vi "Load XCL template.vi"(10 "Measurement template file":path, 11 "Measurement properties":T1={"Measurement frequencies (Hz)"=[1000.0, 10000.0, 1000.0], "Sampling frequency (Hz)"=500000.0, "Signal amplitude (V)"=4.5, "AC-DC settle time (s)"=20.0, "Record length (multiples of period)"=[1000.0, 10000.0, 1000.0], "Measurement template file"=path "", "Row of START keyword"=0, "Row of STOP keyword"=0, "Calculate RMS from samples"=FALSE, "AC-DC warm up time (s)"=300.0} {"Record length (multiples of period)" format="%#_3p"; "Sampling frequency (Hz)" format="%#_3p"; "Measurement frequencies (Hz)" format="%#_3p"}) -> (3 "Measurement properties out":T1={"Measurement frequencies (Hz)"=[1000.0, 10000.0, 1000.0], "Sampling frequency (Hz)"=500000.0, "Signal amplitude (V)"=4.5, "AC-DC settle time (s)"=20.0, "Record length (multiples of period)"=[1000.0, 10000.0, 1000.0], "Measurement template file"=path "", "Row of START keyword"=0, "Row of STOP keyword"=0, "Calculate RMS from samples"=FALSE, "AC-DC warm up time (s)"=300.0} {"Record length (multiples of period)" format="%#_3p"; "Sampling frequency (Hz)" format="%#_3p"; "Measurement frequencies (Hz)" format="%#_3p"})   [LabVIEW 2020]
doc: "Reads values from measurement template in excell spreadsheet."
uses:
  Measurement/Type definitions/Measuement properties.ctl
  <vilib>/Utility/NIReport.llb/Report Type.ctl
  <vilib>/Utility/error.llb/DialogType.ctl
  <vilib>/addons/_office/excel.llb/Excel Get Data ([str]).vi
  <vilib>/Utility/NIReport.llb/NI_report.lvclass
  <vilib>/addons/_office/NI_ReportGenerationToolkit.lvlib
  <vilib>/Utility/NIReport.llb/NI_ReportGenerationCore.lvlib
  <vilib>/Utility/NIReport.llb/Excel/NI_Excel.lvclass
panel:
  out "Stop row":i32
  out "Start row":i32
  out "excell template content":string[][](array[string])
  out "error out":errorcluster
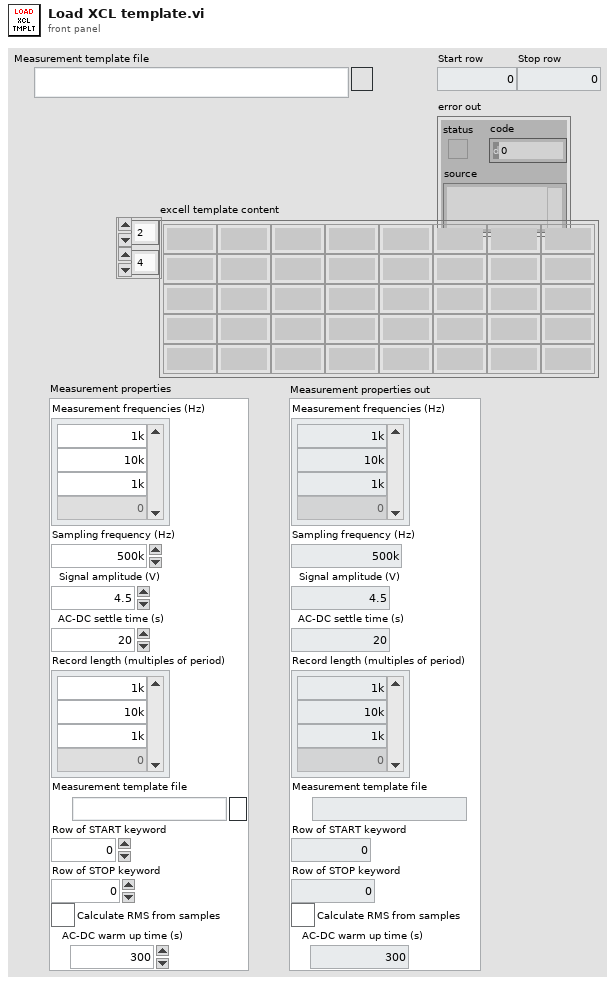
[diagram p1: front panel]
types:
  T1 = typedef "Measuement properties.ctl" = cluster{"Measurement frequencies (Hz)":dbl[], "Sampling frequency (Hz)":dbl, "Signal amplitude (V)":dbl, "AC-DC settle time (s)":dbl, "Record length (multiples of period)":dbl[], "Measurement template file":path, "Row of START keyword":i32, "Row of STOP keyword":i32, "Calculate RMS from samples":bool, "AC-DC warm up time (s)":dbl}
  T2 = enum16{"maximized", "minimized", "normal", "no change"}
  T3 = typedef "NI_ReportGenerationCore.lvlib/Report Type.ctl" = enum16{"HTML", "Word", "Excel"}
  T4 = typedef "DialogType.ctl" = u16
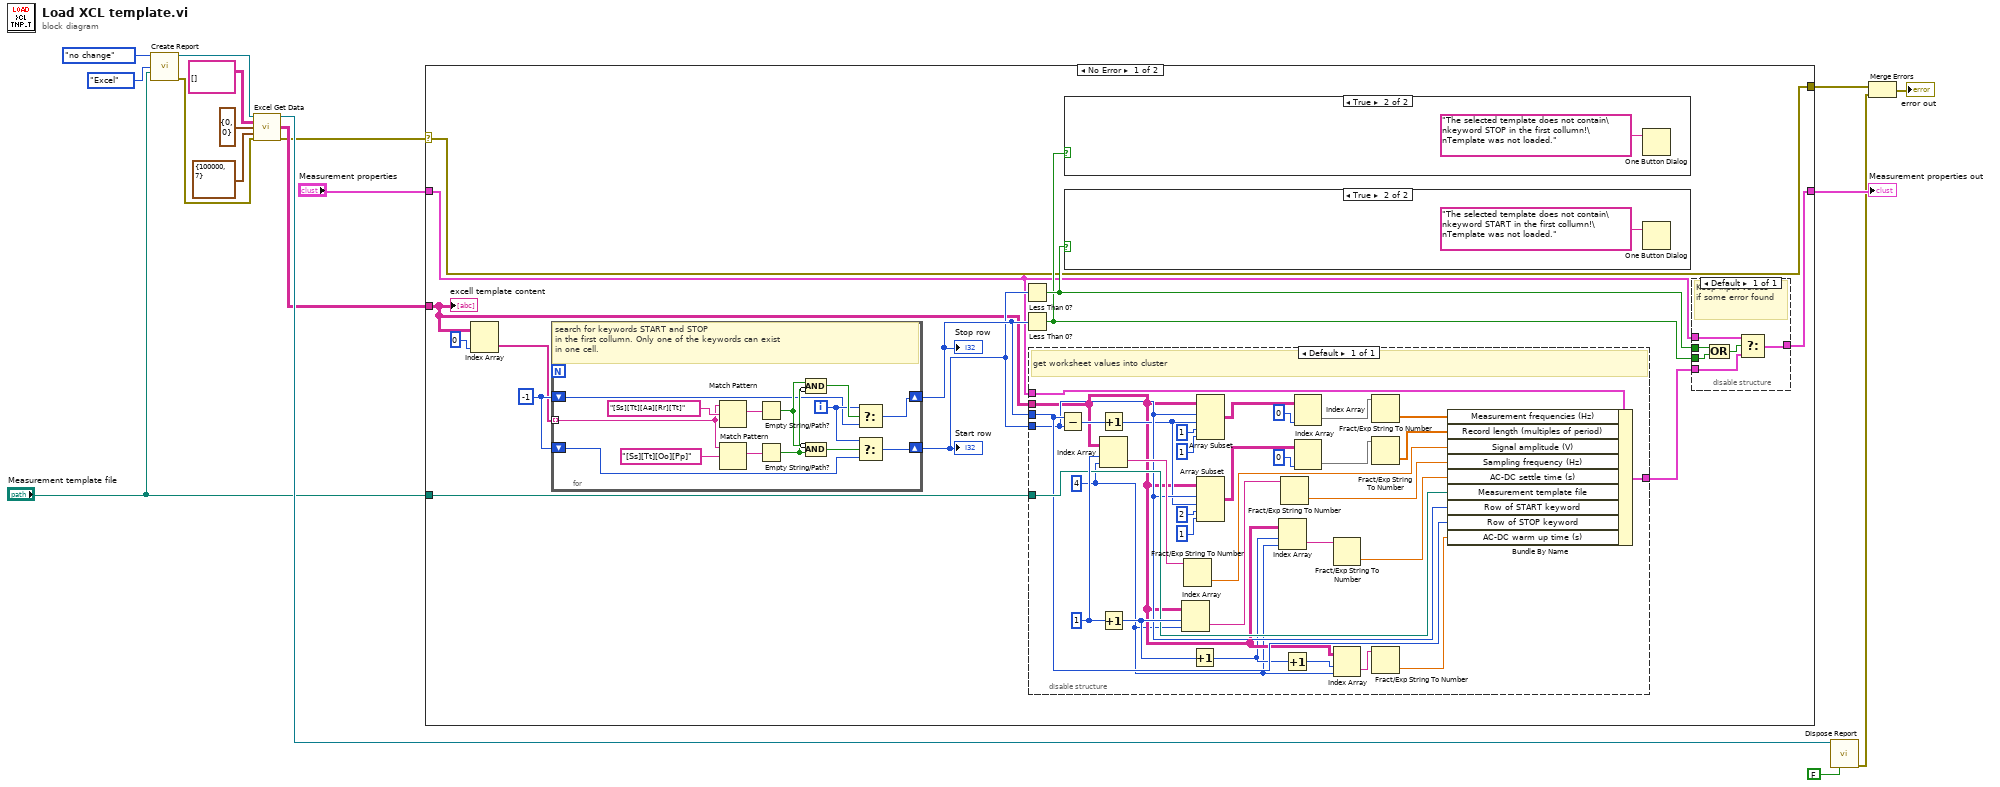
[diagram p0: block diagram]
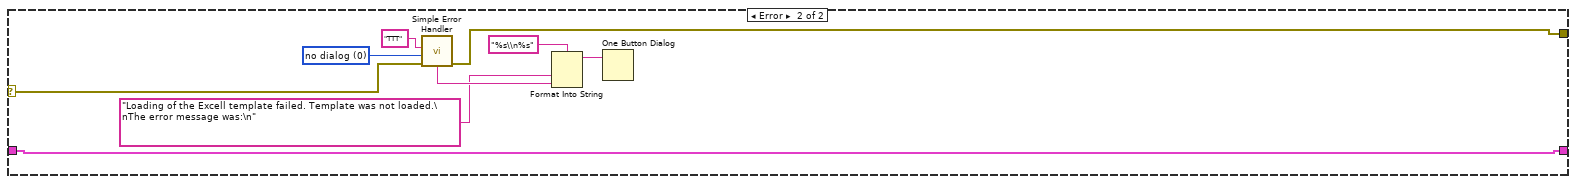
[diagram p4: hidden frame]
diagram:
  n1 = call <vilib>:"Create Report.vi"("window state (normal)"=T2."no change", "report type"=Report_Type."Excel", "template (empty)"="Measurement template file") -> ("report out"=w17:refnum<class "NI_report.lvclass">, "error out"=w16:errorcluster)  [unwired: 11 in]
  n2 = call-poly <vilib>:"Excel Get Data.vi"("report in"=w17, "data type"=string[][] [], "start (-1, -1)"=cluster{"row":i32, "column":i32} {"row"=0, "column"=0}, "end (-1, -1)"=cluster{"row":i32, "column":i32} {"row"=100000, "column"=7}, "error in (no error)"=w16) -> ("report out"=w15:refnum<class "NI_report.lvclass">, "data"=w11:string[][], "error out"=w4:errorcluster)  [unwired: 8 in]
  n3 = case shown="No Error" w4 {
    selector: w4 -> [w18 w93]
    tunnel: w11 -> [w25 _]
    tunnel: [w21 w94] -> w10
    tunnel: "Measurement properties" -> [w20 w94]
    tunnel: "Measurement template file" -> [w19 _]
    tunnel: [w18 w90] -> w3
    frame No Error {
      w29 = -1
      n4 = Index Array(array=w25, index (col)=0 ("disabled index (col)")) -> (element=w28:string[])  [unwired: 1 in]
      n5 = for {
        tunnel: w28 -> [w84] mode=indexing
        shift-right: [w79] -> w26
        shift-left: w29 -> [w72]
        shift-right: [w74] -> w27
        shift-left: w29 -> [w73]
        i -> [w75]
        # "search for keywords START and STOP\nin the first collumn. Only one of the keywords can exist\nin one cell."
        n6 = Match Pattern(string=w84, regular expression="[Ss][Tt][Aa][Rr][Tt]") -> (match substring=w82:string)  [unwired: 1 in, 3 out]
        n7 = Match Pattern(string=w84, regular expression="[Ss][Tt][Oo][Pp]") -> (match substring=w81:string)  [unwired: 1 in, 3 out]
        n8 = Empty String/Path?(string/path=w82) -> (empty?=w78:bool)
        n9 = Empty String/Path?(string/path=w81) -> (empty?=w77:bool)
        n10 = Compound Arithmetic op=AND(w78, invert w77) -> (w76:bool)
        n11 = Compound Arithmetic op=AND(invert w78, w77) -> (w80:bool)
        n12 = Select(t=w75, s=w76, f=w73) -> (s? t:f=w74:i32)
        n13 = Select(t=w75, s=w80, f=w72) -> (s? t:f=w79:i32)
      }
      "Start row" <- w26
      "Stop row" <- w27
      n14 = Less Than 0?(x=w26) -> (x < 0?=w24:bool)
      n15 = Less Than 0?(x=w27) -> (x < 0?=w23:bool)
      n16 = disable-structure shown="Default" {
        disable-tunnel: w27 -> [w46]
        disable-tunnel: w26 -> [w45]
        disable-tunnel: w20 -> [w69]
        disable-tunnel: w25 -> [w41]
        disable-tunnel: [w62] -> w22
        disable-tunnel: w19 -> [w47]
        frame Enabled {
          w38 = 4 ("index")
          w53 = 1 ("index")
          # "get worksheet values into cluster"
          n17 = Subtract(x=w46, y=w45) -> (x-y=w44:i32)
          n18 = Increment(x=w44) -> (x+1=w43:i32)
          n19 = Index Array(array=w41, index (row)=w53, index (col)=w38) -> (element=w55:string)
          n20 = Increment(x=w53) -> (x+1=w49:i32)
          n21 = Index Array(array=w41, index (row)=w49, index (col)=w38) -> (element=w52:string)
          n22 = Fract/Exp String To Number(string=w55) -> (number=w54:dbl)  [unwired: 3 in, 1 out]
          n23 = Increment(x=w49) -> (x+1=w39:i32)
          n24 = Array Subset(array=w41, index (row)=w45, length (row)=w43, index (col)=1 ("index"), length (col)=1 ("length")) -> (w66:string[][])
          n25 = Array Subset(array=w41, index (row)=w45, length (row)=w43, index (col)=2 ("index"), length (col)=1 ("length")) -> (w59:string[][])
          n26 = Index Array(array=w41, index (row)=w39, index (col)=w38) -> (element=w50:string)
          n27 = Fract/Exp String To Number(string=w52) -> (number=w51:dbl)  [unwired: 3 in, 1 out]
          n28 = Increment(x=w39) -> (x+1=w40:i32)
          n29 = Index Array(array=w66, index (col)=0 ("index (row)")) -> (element=w64:string[])  [unwired: 1 in]
          n30 = Index Array(array=w59, index (col)=0 ("index (row)")) -> (element=w61:string[])  [unwired: 1 in]
          n31 = Fract/Exp String To Number(string=w50) -> (number=w48:dbl)  [unwired: 3 in, 1 out]
          n32 = Index Array(array=w41, index (row)=w40, index (col)=w38) -> (element=w42:string)
          n33 = Fract/Exp String To Number(string=w64) -> (number=w63:dbl[])  [unwired: 3 in, 1 out]
          n34 = Fract/Exp String To Number(string=w61) -> (number=w56:dbl[])  [unwired: 3 in, 1 out]
          n35 = Fract/Exp String To Number(string=w42) -> (number=w37:dbl)  [unwired: 3 in, 1 out]
          n36 = Bundle By Name(cluster=w69, "Measurement frequencies (Hz)"=w63, "Record length (multiples of period)"=w56, "Signal amplitude (V)"=w54, "Sampling frequency (Hz)"=w51, "AC-DC settle time (s)"=w48, "Measurement template file"=w47, "Row of START keyword"=w45, "Row of STOP keyword"=w46, "AC-DC warm up time (s)"=w37) -> (w62:T1)
        }
      }
      n37 = case shown="True" w23 {
        frame False {
        }
        frame True {
          n38 = One Button Dialog(message="The selected template does not contain\nkeyword STOP in the first collumn!\nTemplate was not loaded.") -> ()  [unwired: 1 in, 1 out]
        }
      }
      n39 = case shown="True" w24 {
        frame False {
        }
        frame True {
          n40 = One Button Dialog(message="The selected template does not contain\nkeyword START in the first collumn!\nTemplate was not loaded.") -> ()  [unwired: 1 in, 1 out]
        }
      }
      n41 = disable-structure shown="Default" {
        disable-tunnel: w24 -> [w35]
        disable-tunnel: w23 -> [w34]
        disable-tunnel: w22 -> [w33]
        disable-tunnel: [w32] -> w21
        disable-tunnel: w20 -> [w31]
        frame Enabled {
          # "Keep input values\nif some error found"
          n42 = Compound Arithmetic op=OR(w35, w34) -> (w36:bool)
          n43 = Select(t=w31, s=w36, f=w33) -> (s? t:f=w32:T1)
        }
      }
      "excell template content" <- w25
    }
    frame Error {
      w92 = T4 0 items=["no dialog", "OK message", "continue or stop message", "OK message + warnings", "continue/stop + warnings"] ("type of dialog (OK msg:1)")
      n44 = call <vilib>:"Simple Error Handler.vi"("error source (\" \")"="TTT" ("error source (\" \")"), "type of dialog (OK msg:1)"=w92, "error in (no error)"=w93) -> ("error out"=w90:errorcluster, "message"=w87:string)  [unwired: 2 in, 3 out]
      n45 = Format Into String(format string="%s\\n%s", "Loading of the Excell template failed. Template was not loaded.\nThe error message was:\n" ("input 1"), w87) -> (resulting string=w88:string)  [unwired: 2 in, 1 out]
      n46 = One Button Dialog(message=w88) -> ()  [unwired: 1 in, 1 out]
    }
  }
  "Measurement properties out" <- w10
  n47 = call-dynamic "Dispose Report.vi"("report in"=w15, "close report? (T)"=FALSE) -> ("error out"=w2:errorcluster)  [unwired: 13 in]
  n48 = Merge Errors(w3, w2) -> (→"error out":errorcluster)
